vi "xPCOpenTcpIpPort.vi"(2 "port":string, 3 "address":string) -> (0 "error out":errorcluster, 1 "Port":i32)   [LabVIEW 2018]
uses:
  XPCAPI.DLL
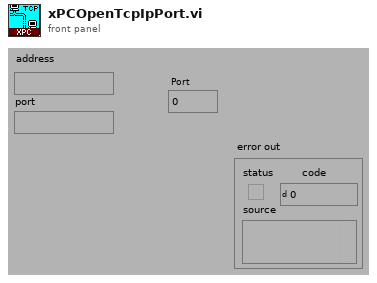
[diagram p1: front panel]
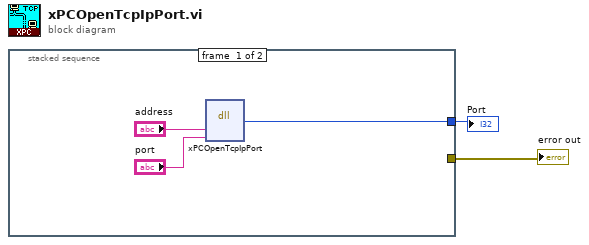
[diagram p0: block diagram]
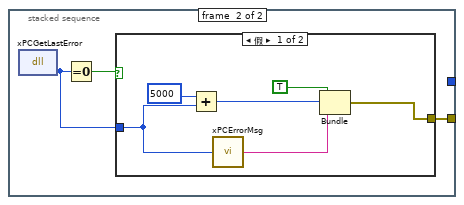
[diagram p2: hidden frame]
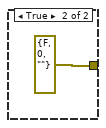
[diagram p3: hidden frame]
diagram:
  n1 = stacked-sequence {
    tunnel: [w3 _] -> w1
    tunnel: [_ w6] -> w2
    frame #0 {
      n2 = dll-call lib="PTH2Cabs CUserszczgDesktop上下位机联机测试\nxpcapi.dll" fn="xPCOpenTcpIpPort"("address"="address", "port"="port") -> (w3:i32)  [unwired: 5 in, 2 out]
    }
    frame #1 {
      n3 = dll-call lib="PTH2Cabs CUserszczgDesktop上下位机联机测试\nxpcapi.dll" fn="xPCGetLastError"() -> (w7:i32)  [unwired: 3 in, 2 out]
      n4 = Equal To 0?(x=w7) -> (x = 0?=w8:bool)
      n5 = case shown="假" w8 {
        tunnel: w7 -> [w10 _]
        tunnel: [w11 errorcluster {"status"=FALSE, "code"=0, "source"=""} ("error out")] -> w6
        frame False {
          n6 = Add(x=5000 ("y"), y=w10) -> (x+y=w13:i32)
          n7 = call "xPCErrorMsg.vi"("error number"=w10) -> ("ErrorMsg"=w12:string)
          n8 = Bundle(TRUE, w13, "ErrorMsg"=w12) -> (w11:cluster{bool, i32, "ErrorMsg":string})  [unwired: 1 in]
        }
        frame True {
        }
      }
    }
  }
  "error out" <- w2
  "Port" <- w1
